vi "Set Numbers And Operations On Instances.vi"(8 "error in (no error)":errorcluster, 10 "Operations":T1(array[cluster]), 11 "Array":refnum<class "SimpleArithmetic.lvclass">[](array[class])) -> (0 "error out":errorcluster, 3 "Array Out":refnum<class "SimpleArithmetic.lvclass">[](array[class]))   [LabVIEW 2013]
uses:
  ClassDefinitions/SimpleClassWithMethods/SimpleArithmetic.lvclass
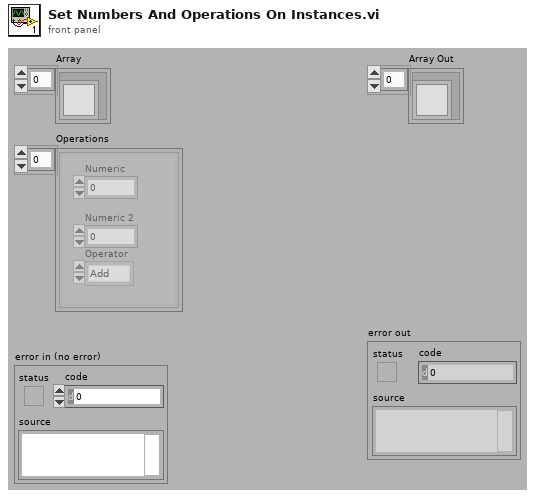
[diagram p1: front panel]
types:
  T1 = cluster{"Numeric":dbl, "Numeric 2":dbl, "Operator":enum16{"Add", "Divide", "Multiple", "Subtract"}}[]
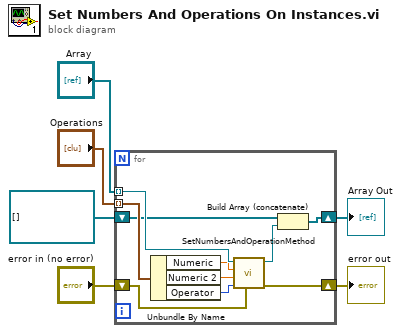
[diagram p0: block diagram]
diagram:
  n1 = for {
    tunnel: "Array" -> [w16] mode=indexing
    tunnel: "Operations" -> [w15] mode=indexing
    shift-right: [w7] -> w1
    shift-left: refnum<class "SimpleArithmetic.lvclass">[] [] ("Array") -> [w10]
    shift-right: [w8] -> w2
    shift-left: "error in (no error)" -> [w11]
    n2 = Unbundle By Name(w15) -> ("Numeric"=w14:dbl, "Numeric 2"=w13:dbl, "Operator"=w12:enum16{"Add", "Divide", "Multiple", "Subtract"})
    n3 = call "SetNumbersAndOperationMethod.vi"("error in (no error)"=w11, "Operator"=w12, "Numeric 2"=w13, "Numeric"=w14, "SimpleArithmetic in"=w16) -> ("error out"=w8:errorcluster, "SimpleArithmetic out"=w9:refnum<class "SimpleArithmetic.lvclass">)  [unwired: 5 in]
    n4 = Build Array (concatenate)(w10, w9) -> (w7:refnum<class "SimpleArithmetic.lvclass">[])
  }
  "Array Out" <- w1
  "error out" <- w2
